vi "SPI Read Bits.vi"(7 "ReadBitsNum":i32, 9 "pReadBitStr":u8[](array[numeric])=array[4097 elements], 10 "SPIIndex":i32, 11 "DevHandle":i32) -> (1 "pReadBitStr out":u8[](array[numeric]), 3 "function return":i32)   [LabVIEW 2010, in "usb2spi.lvlib"]
doc: "int WINAPI SPI_ReadBits(int DevHandle,int SPIIndex,char *pReadBitStr,int ReadBitsNum);"
uses:
  usb2spi.lvlib
  USB2XXX/trunk/USB2XXX/USB2XXX/vs2019/Release/USB2XXX.dll
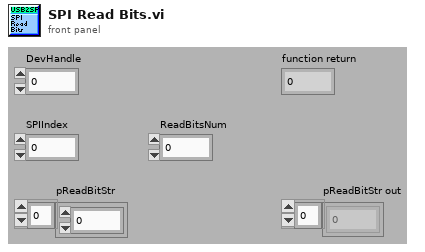
[diagram p1: front panel]
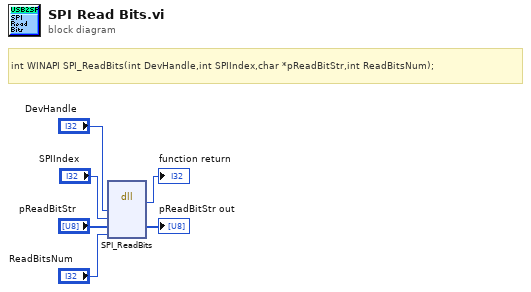
[diagram p0: block diagram]
diagram:
  # "int WINAPI SPI_ReadBits(int DevHandle,int SPIIndex,char *pReadBitStr,int ReadBitsNum);"
  n1 = dll-call lib="E:/Projects/USB2XXX/trunk/USB2XXX/USB2XXX/vs2019/Release/USB2XXX.*" fn="SPI_ReadBits"("DevHandle"="DevHandle", "SPIIndex"="SPIIndex", "pReadBitStr"="pReadBitStr", "ReadBitsNum"="ReadBitsNum") -> (→"function return":i32, "pReadBitStr"=→"pReadBitStr out":u8[])  [unwired: 6 in, 2 out]
